vi "GetOrigDlyDist.vi"(8 "错误输入（无错误）":errorcluster, 11 "Chan":u8) -> (0 "错误输出":errorcluster, 3 "返回值":sgl)   [LabVIEW 2014]
uses:
  X86Dll/ZXUTConfigMgr.dll
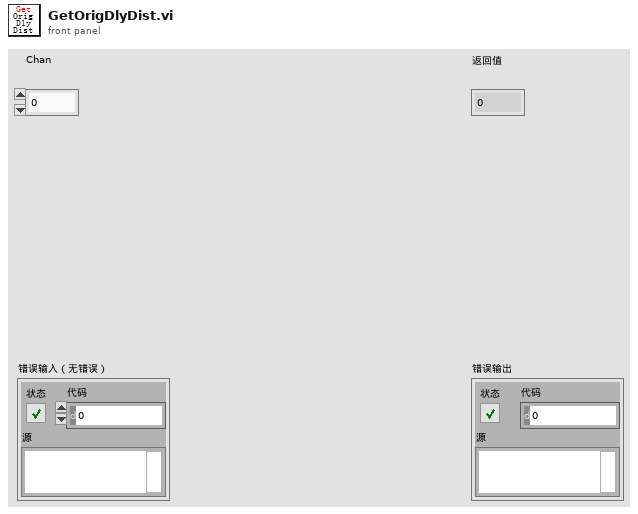
[diagram p1: front panel]
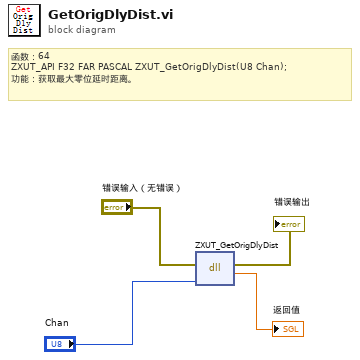
[diagram p0: block diagram]
diagram:
  # "函数：64\nZXUT_API F32\tFAR PASCAL ZXUT_GetOrigDlyDist(U8 Chan);\n功能：获取最大零位延时距离。"
  n1 = dll-call lib="D:/Software/Utrasonic on-line monitoring/X86Dll/ZXUTConfigMgr.dll" fn="ZXUT_GetOrigDlyDist"(error in="错误输入（无错误）", "Chan"="Chan") -> (error out=→"错误输出":errorcluster, "返回值"=→"返回值":sgl)  [unwired: 3 in, 1 out]
